vi "Wfm odczytaj ustawienia.vi"(8 "error in (no error)":errorcluster, 11 "Wfm Refs in":refnum<vi>[](array[refnum])) -> (0 "error out":errorcluster, 3 "Wfm Refs out":refnum<vi>[](array[refnum]), 4 "Plot Bounds":T1[](array[typedef]), 5 "Plot Area Widths":u32[](array[numeric]), 6 "NO skale":bool[][](array[boolean]))   [LabVIEW 2014]
doc: "odczytuje z wykresów\naktywne skale oraz rozmiary i pozycje elementów komponentu"
uses:
  <vilib>/Utility/miscctls.llb/LVRectTypeDef.ctl
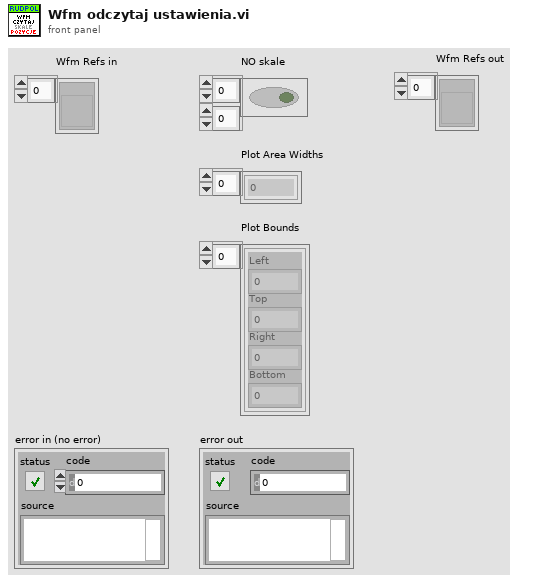
[diagram p1: front panel]
types:
  T1 = typedef "LVRectTypeDef.ctl" = cluster{"Left":i16, "Top":i16, "Right":i16, "Bottom":i16}
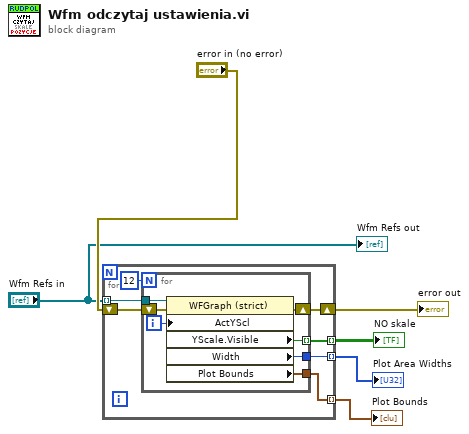
[diagram p0: block diagram]
diagram:
  n1 = for {
    tunnel: "Wfm Refs in" -> [w13] mode=indexing
    tunnel: [w11] -> w2 mode=indexing
    shift-right: [w9] -> w4
    shift-left: "error in (no error)" -> [w10]
    tunnel: [w8] -> w3 mode=indexing
    tunnel: [w7] -> w5 mode=indexing
    n2 = for {
      N: 12 -> [_]
      tunnel: w13 -> [w20]
      tunnel: [w18] -> w11 mode=indexing
      shift-right: [w16] -> w9
      shift-left: w10 -> [w17]
      tunnel: [w15] -> w8
      tunnel: [w14] -> w7
      i -> [w19]
      n3 = property class="WFGraph (strict)"(reference=w20, error in=w17, "ActYScl"=w19) -> (error out=w16:errorcluster, "YScale.Visible"=w18:bool, "Width"=w15:u32, "Plot Bounds"=w14:T1)  [unwired: 1 out]
    }
  }
  "Plot Bounds" <- w5
  "error out" <- w4
  "Plot Area Widths" <- w3
  "NO skale" <- w2
  "Wfm Refs out" <- "Wfm Refs in"
